vi "ConsumeTransform.vi"(8 "error in (no error)":errorcluster, 11 "TransformTokenizer in":refnum<class "TransformTokenizer.lvclass">) -> (0 "error out":errorcluster, 3 "TransformTokenizer out":refnum<class "TransformTokenizer.lvclass">)   [LabVIEW 2019, in "TransformTokenizer.lvclass"]
uses:
  TransformTokenizer.lvclass
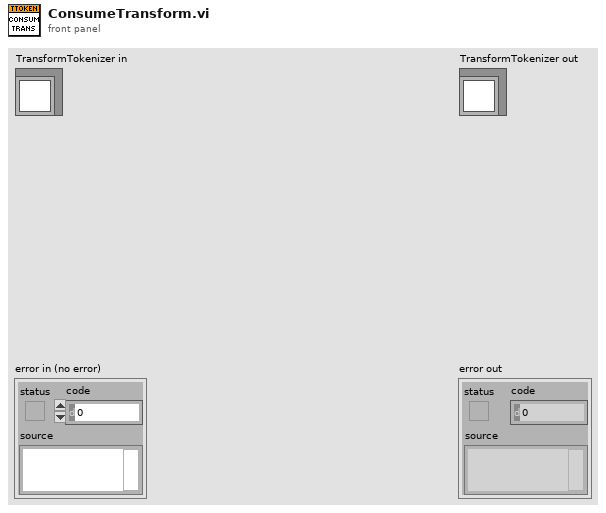
[diagram p1: front panel]
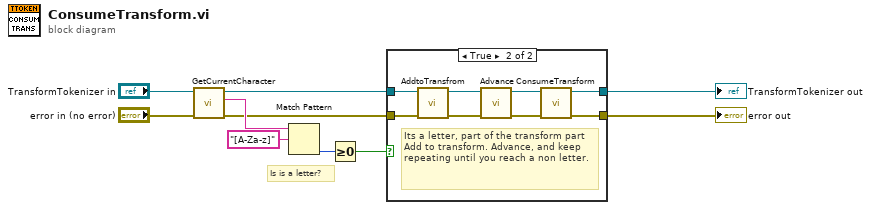
[diagram p0: block diagram]
diagram:
  # "Is is a letter?"
  n1 = call "GetCurrentCharacter.vi"("error in (no error)"="error in (no error)", "TransformTokenizer in"="TransformTokenizer in") -> ("error out"=w3:errorcluster, "Character"=w9:string, "TransformTokenizer out"=w5:refnum<class "TransformTokenizer.lvclass">)  [unwired: 7 in]
  n2 = Match Pattern(string=w9, regular expression="[A-Za-z]") -> (offset past match=w6:i32)  [unwired: 1 in, 3 out]
  n3 = Greater Or Equal To 0?(x=w6) -> (x >= 0?=w1:bool)
  n4 = case shown="True" w1 {
    tunnel: w5 -> [w12 w20]
    tunnel: [w12 w15] -> w4
    tunnel: w3 -> [w11 w19]
    tunnel: [w11 w13] -> w2
    frame False {
    }
    frame True {
      # "Its a letter, part of the transform part\nAdd to transform. Advance, and keep repeating until you reach a non letter."
      n5 = call "AddtoTransfrom.vi"("error in (no error)"=w19, "TransformTokenizer in"=w20) -> ("error out"=w17:errorcluster, "TransformTokenizer out"=w18:refnum<class "TransformTokenizer.lvclass">)  [unwired: 8 in]
      n6 = call "Advance.vi"("error in (no error)"=w17, "TransformTokenizer in"=w18) -> ("error out"=w14:errorcluster, "TransformTokenizer out"=w16:refnum<class "TransformTokenizer.lvclass">)  [unwired: 8 in]
      n7 = call "ConsumeTransform.vi"("error in (no error)"=w14, "TransformTokenizer in"=w16) -> ("error out"=w13:errorcluster, "TransformTokenizer out"=w15:refnum<class "TransformTokenizer.lvclass">)  [unwired: 8 in]
    }
  }
  "error out" <- w2
  "TransformTokenizer out" <- w4
